vi "run.vi"(8 "error in (no error)":errorcluster, 10 "test":refnum<class>, 11 "TextTestRunner in":refnum<class "TextTestRunner.lvclass">) -> (0 "error out":errorcluster, 3 "TextTestRunner out":refnum<class "TextTestRunner.lvclass">)   [LabVIEW 2009, in "TextTestRunner.lvclass"]
uses:
  TextTestRunner.lvclass
  TestCase/TestCase.lvclass
  TextTestRunner.lvclass/TextTestRunner.ctl
  TestSuite/TestSuite.lvclass
  _TextTestResult/_TextTestResult.lvclass
panel:
  # "JKI VI Tester for LabVIEW\nhttp://jkisoft.com/vi-tester\nCopyright (C) 2007-2009, JKI <info@jkisoft.com>\nALL RIGHTS RESERVED"
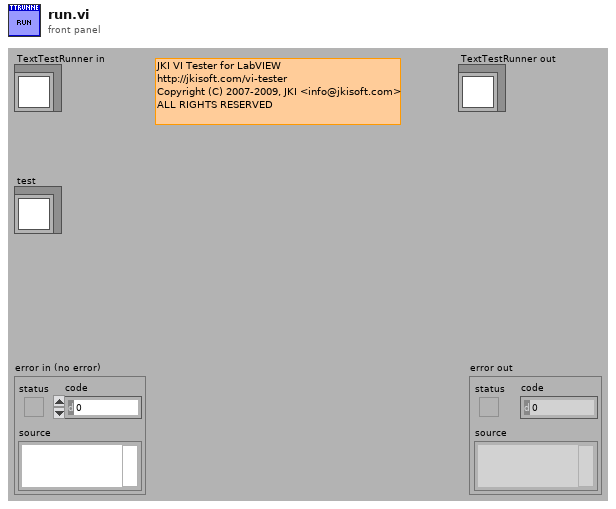
[diagram p1: front panel]
types:
  T1 = typedef "TestResult.lvclass/failure.ctl" = cluster{"test":refnum<class>, "error":errorcluster}
  T2 = typedef "TestResult.lvclass/errors.ctl" = T3[]
  T3 = typedef "TestResult.lvclass/error.ctl" = cluster{"test":refnum<class>, "error":errorcluster}
  T4 = typedef "TestResult.lvclass/skipped.ctl" = T5[]
  T5 = typedef "TestResult.lvclass/skip.ctl" = cluster{"test":refnum<class>, "error":errorcluster}
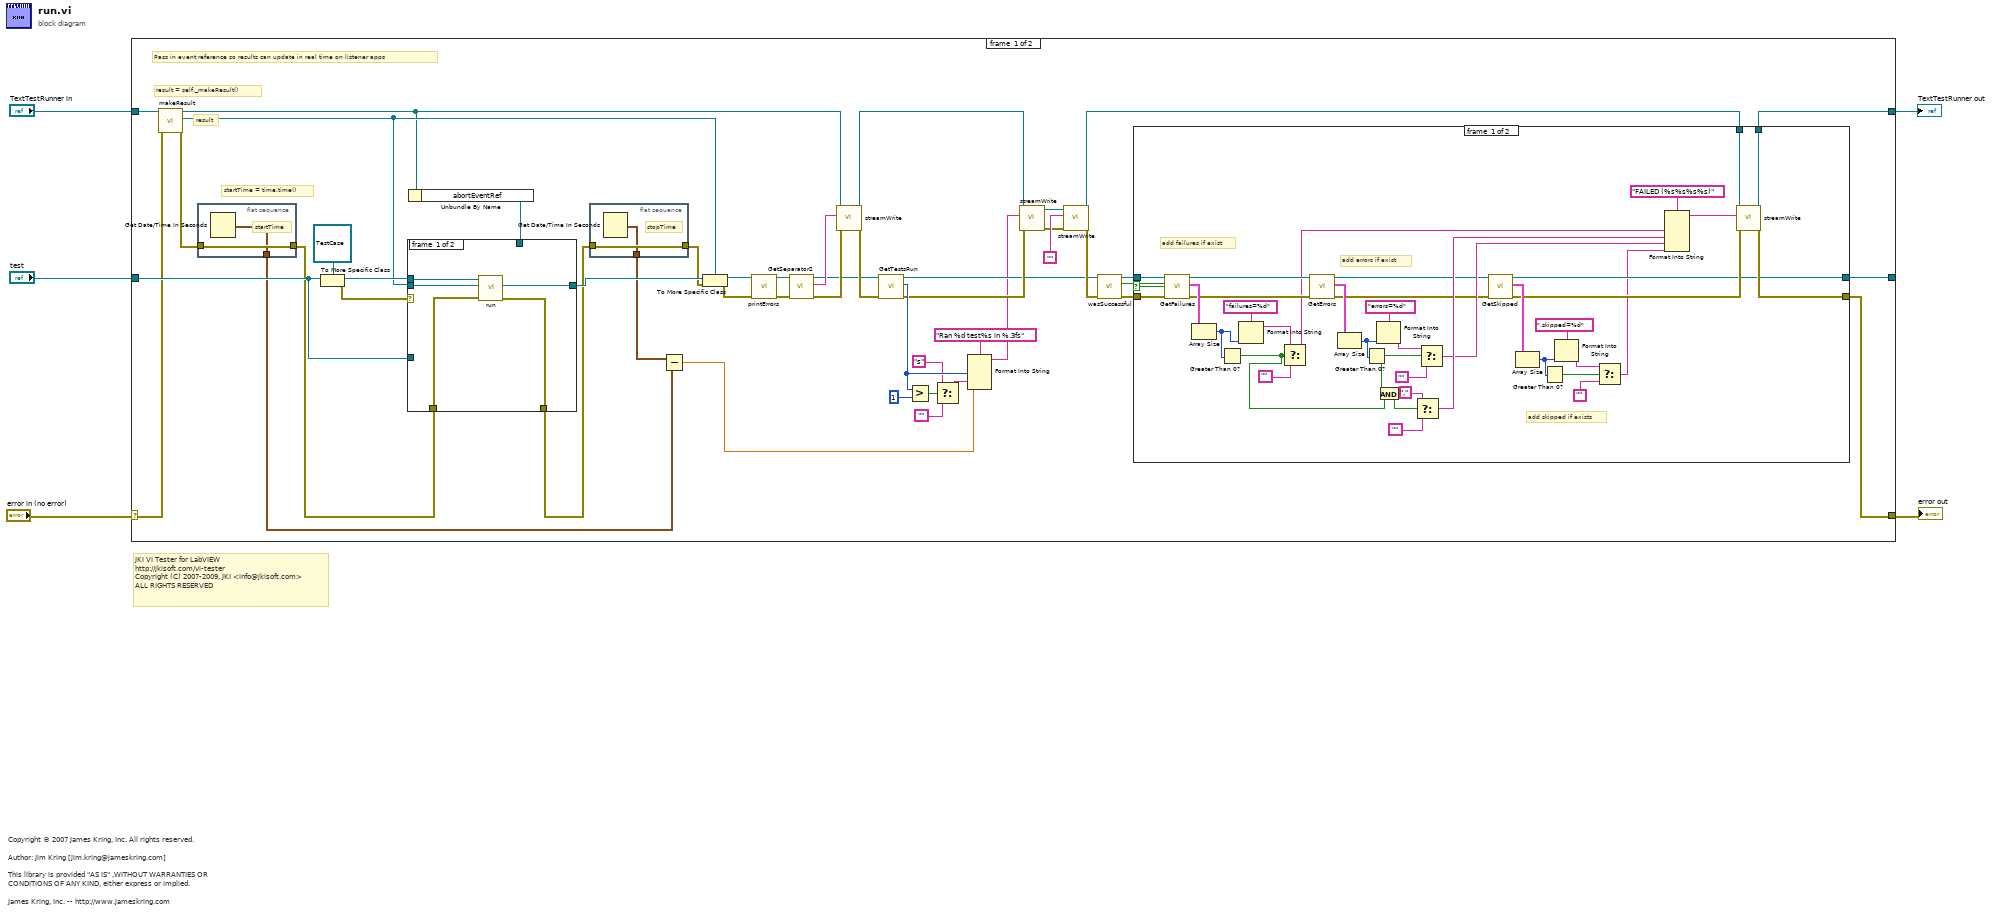
[diagram p0: block diagram]
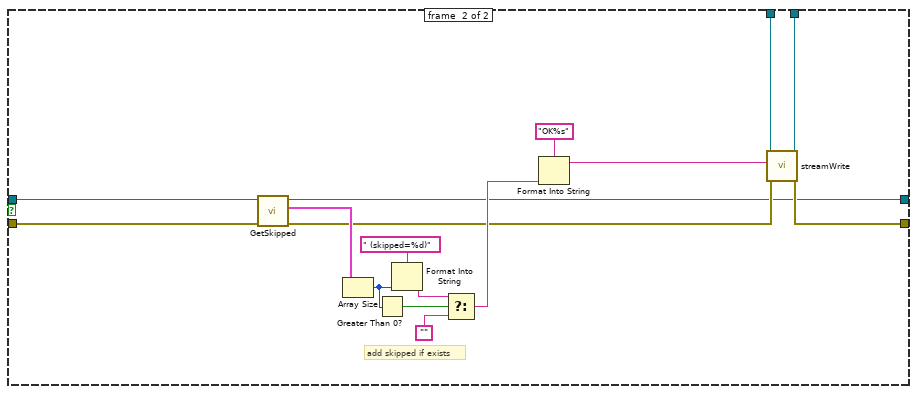
[diagram p2: hidden frame]
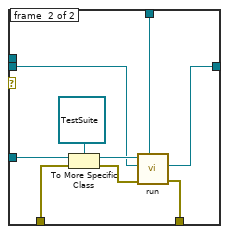
[diagram p3: hidden frame]
diagram:
  # "JKI VI Tester for LabVIEW\nhttp://jkisoft.com/vi-tester\nCopyright (C) 2007-2009, JKI <info@jkisoft.com>\nALL RIGHTS RESERVED"
  # "Copyright © 2007 James Kring, Inc. All rights reserved.\n\nAuthor: Jim Kring [jim.kring@jameskring.com]\n\nThis library is provided \"AS IS\" ,WITHOUT WARRANTIES OR \nCONDITIONS OF ANY KIND, either express or implied.\n\nJames Kring, Inc. -- http://www.jameskring.com"
  n1 = case shown="No Error" "error in (no error)" {
    selector: "error in (no error)" -> [w47 w126]
    tunnel: [w27 w126] -> w4
    tunnel: [w12 w125] -> w2
    tunnel: "TextTestRunner in" -> [w52 w125]
    tunnel: "test" -> [w48 _]
    tunnel: [w26 _] -> _
    frame #0 {
      # "Pass in event reference so results can update in real time on listener apps"
      # "startTime = time.time()"
      # "result"
      # "result = self._makeResult()"
      n2 = call-dynamic "makeResult.vi"("error in (no error)"=w47, "TextTestRunner in"=w52) -> ("error out"=w43:errorcluster, "TestTestResult"=w45:refnum<class "_TextTestResult.lvclass">, "TextTestRunner out"=w7:refnum<class "TextTestRunner.lvclass">)  [unwired: 7 in]
      n3 = flat-sequence {
        tunnel: [w110] -> w44
        tunnel: w43 -> [w110]
        tunnel: [w109] -> w38
        frame #0 {
          # "startTime"
          n4 = Get Date/Time In Seconds() -> (seconds since 1Jan1904=w109:timestamp)
        }
      }
      n5 = To More Specific Class(target class=refnum<class "TestCase.lvclass"> refnum ("TestCase in"), reference=w48) -> (specific class reference=w50:refnum<class "TestCase.lvclass">, error out=w49:errorcluster)  [unwired: 1 in]
      n6 = Unbundle By Name(w7) -> ("abortEventRef"=w6:refnum<user-event>)
      n7 = case shown="Error" w49 {
        tunnel: w50 -> [w111 _]
        tunnel: w45 -> [w112 w118]
        tunnel: w48 -> [_ w124]
        tunnel: w44 -> [w115 w120]
        tunnel: [w114 w121] -> w42
        tunnel: [w113 w117] -> w46
        tunnel: w6 -> [_ w116]
        frame #0 {
          n8 = call "run.vi"("error in (no error)"=w115, "TestResult in (None: Create New)"=w112, "TestCase in"=w111) -> ("error out"=w114:errorcluster, "TestResult out"=w113:refnum<class "TestResult.lvclass">)  [unwired: 6 in, 1 out]
        }
        frame #1 {
          n9 = To More Specific Class(target class=refnum<class "TestSuite.lvclass"> refnum ("reference in"), reference=w124, error in=w120) -> (specific class reference=w122:refnum<class "TestSuite.lvclass">, error out=w119:errorcluster)
          n10 = call "run.vi"("abortEvent"=w116, "error in (no error)"=w119, "TestResult in"=w118, "TestSuite in"=w122) -> ("error out"=w121:errorcluster, "TestResult out"=w117:refnum<class "TestResult.lvclass">)  [unwired: 5 in, 1 out]
        }
      }
      n11 = flat-sequence {
        tunnel: [w108] -> w41
        tunnel: w42 -> [w108]
        tunnel: [w107] -> w39
        frame #0 {
          # "stopTime"
          n12 = Get Date/Time In Seconds() -> (seconds since 1Jan1904=w107:timestamp)
        }
      }
      n13 = Subtract(x=w39, y=w38) -> (x-y=w37:dbl)
      n14 = To More Specific Class(target class=w45, reference=w46, error in=w41) -> (specific class reference=w11:refnum<class "_TextTestResult.lvclass">, error out=w8:errorcluster)
      n15 = call-dynamic "printErrors.vi"("error in (no error)"=w8, "TestTestResult in"=w11) -> ("error out"=w10:errorcluster, "TestTestResult out"=w9:refnum<class "_TextTestResult.lvclass">)  [unwired: 8 in]
      n16 = call-dynamic "GetSeparator2.vi"("error in (no error)"=w10, "TestTestResult in"=w9) -> ("error out"=w24:errorcluster, "separator2"=w25:string, "TestTestResult out"=w22:refnum<class "_TextTestResult.lvclass">)  [unwired: 7 in]
      n17 = call-dynamic "streamWrite.vi"("error in (no error)"=w24, "String"=w25, "TextTestRunner in"=w7) -> ("error out"=w23:errorcluster, "TextTestRunner out"=w15:refnum<class "TextTestRunner.lvclass">)  [unwired: 7 in]
      n18 = call-dynamic "GetTestsRun.vi"("error in (no error)"=w23, "TestResult in"=w22) -> ("error out"=w20:errorcluster, "testsRun"=w36:u32, "TestResult out"=w17:refnum<class "_TextTestResult.lvclass">)  [unwired: 7 in]
      n19 = Greater?(x=w36, y=u32 1) -> (0:w34:bool)
      n20 = Select(t="s", s=w34, f="") -> (s? t:f=w31:string)
      n21 = Format Into String(format string="Ran %d test%s in %.3fs", w36, w31, w37) -> (resulting string=w16:string)  [unwired: 2 in, 1 out]
      n22 = call-dynamic "streamWrite.vi"("error in (no error)"=w20, "String"=w16, "TextTestRunner in"=w15) -> ("error out"=w19:errorcluster, "TextTestRunner out"=w14:refnum<class "TextTestRunner.lvclass">)  [unwired: 7 in]
      n23 = call-dynamic "streamWrite.vi"("error in (no error)"=w19, "String"="", "TextTestRunner in"=w14) -> ("error out"=w18:errorcluster, "TextTestRunner out"=w13:refnum<class "TextTestRunner.lvclass">)  [unwired: 7 in]
      n24 = call-dynamic "wasSuccessful.vi"("error in (no error)"=w18, "TestResult in"=w17) -> ("error out"=w28:errorcluster, "successful?"=w30:bool, "TestResult in"=w29:refnum<class "_TextTestResult.lvclass">)  [unwired: 7 in]
      n25 = case shown="True" w30 {
        tunnel: w29 -> [w69 w92]
        tunnel: w28 -> [w68 w94]
        tunnel: [w56 w91] -> w26
        tunnel: [w64 w104] -> w27
        tunnel: w13 -> [w67 w106]
        tunnel: [w66 w105] -> w12
        frame #0 {
          # "add errors if exist"
          # "add failures if exist"
          # "add skipped if exists"
          n26 = call-dynamic "GetFailures.vi"("error in (no error)"=w68, "TestResult in"=w69) -> ("error out"=w78:errorcluster, "failures"=w90:T1[], "TestResult out"=w79:refnum<class "_TextTestResult.lvclass">)  [unwired: 7 in]
          n27 = Array Size(array=w90) -> (size(s)=w88:i32)
          n28 = Greater Than 0?(x=w88) -> (x > 0?=w75:bool)
          n29 = Format Into String(format string="failures=%d" ("String"), w88) -> (resulting string=w87:string)  [unwired: 2 in, 1 out]
          n30 = Select(t=w87, s=w75, f="") -> (s? t:f=w72:string)
          n31 = call-dynamic "GetErrors.vi"("error in (no error)"=w78, "TestResult in"=w79) -> ("error out"=w59:errorcluster, "Errors"=w84:T2, "TestResult out"=w57:refnum<class "_TextTestResult.lvclass">)  [unwired: 7 in]
          n32 = Array Size(array=w84) -> (size(s)=w82:i32)
          n33 = Greater Than 0?(x=w82) -> (x > 0?=w76:bool)
          n34 = Format Into String(format string="errors=%d" ("String"), w82) -> (resulting string=w80:string)  [unwired: 2 in, 1 out]
          n35 = And(x=w76, y=w75) -> (x .and. y?=w74:bool)
          n36 = Select(t=",", s=w74, f="") -> (s? t:f=w71:string)
          n37 = Select(t=w80, s=w76, f="") -> (s? t:f=w70:string)
          n38 = call-dynamic "GetSkipped.vi"("error in (no error)"=w59, "TestResult in"=w57) -> ("error out"=w58:errorcluster, "Skipped"=w60:T4, "TestResult in"=w56:refnum<class "_TextTestResult.lvclass">)  [unwired: 7 in]
          n39 = Array Size(array=w60) -> (size(s)=w61:i32)
          n40 = Greater Than 0?(x=w61) -> (x > 0?=w63:bool)
          n41 = Format Into String(format string=",skipped=%d" ("String"), w61) -> (resulting string=w62:string)  [unwired: 2 in, 1 out]
          n42 = Select(t=w62, s=w63, f="") -> (s? t:f=w53:string)
          n43 = Format Into String(format string="FAILED (%s%s%s%s)" ("String"), w72, w71, w70, w53) -> (resulting string=w65:string)  [unwired: 2 in, 1 out]
          n44 = call-dynamic "streamWrite.vi"("error in (no error)"=w58, "String"=w65, "TextTestRunner in"=w67) -> ("error out"=w64:errorcluster, "TextTestRunner out"=w66:refnum<class "TextTestRunner.lvclass">)  [unwired: 7 in]
        }
        frame #1 {
          # "add skipped if exists"
          n45 = call-dynamic "GetSkipped.vi"("error in (no error)"=w94, "TestResult in"=w92) -> ("error out"=w93:errorcluster, "Skipped"=w100:T4, "TestResult in"=w91:refnum<class "_TextTestResult.lvclass">)  [unwired: 7 in]
          n46 = Array Size(array=w100) -> (size(s)=w101:i32)
          n47 = Greater Than 0?(x=w101) -> (x > 0?=w103:bool)
          n48 = Format Into String(format string=" (skipped=%d)" ("String"), w101) -> (resulting string=w102:string)  [unwired: 2 in, 1 out]
          n49 = Select(t=w102, s=w103, f="") -> (s? t:f=w96:string)
          n50 = Format Into String(format string="OK%s", w96) -> (resulting string=w95:string)  [unwired: 2 in, 1 out]
          n51 = call-dynamic "streamWrite.vi"("error in (no error)"=w93, "String"=w95, "TextTestRunner in"=w106) -> ("error out"=w104:errorcluster, "TextTestRunner out"=w105:refnum<class "TextTestRunner.lvclass">)  [unwired: 7 in]
        }
      }
    }
    frame #1 {
    }
  }
  "error out" <- w4
  "TextTestRunner out" <- w2
